vi "Cleanup.vi"(8 "error in (no error)":errorcluster, 11 "OBS in":refnum<class "OBS.lvclass">) -> (0 "error out":errorcluster)   [LabVIEW 2020, in "obs-websocket.lvlib" / "OBS.lvclass"]
uses:
  OBS.lvclass
  Command.ctl
  OBS.lvclass/OBS.ctl
  lv-promises/Promises/Promise/Promise.lvclass
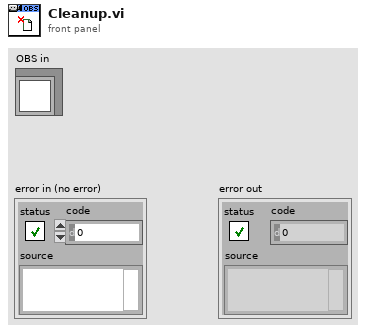
[diagram p1: front panel]
types:
  T1 = typedef "obs-websocket.lvlib/OBS.lvclass/Command.ctl" = enum16{"Open", "Close", "Stop"}
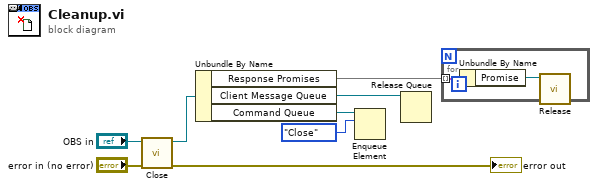
[diagram p0: block diagram]
diagram:
  n1 = call "Close.vi"("error in (no error)"="error in (no error)", "OBS in"="OBS in") -> ("error out"=→"error out":errorcluster, "OBS out"=w6:refnum<class "OBS.lvclass">)  [unwired: 8 in]
  n2 = Unbundle By Name(w6) -> ("Response Promises"=w1:map{string, refnum<class "Promise.lvclass">}, "Client Message Queue"=w5:refnum<queue>, "Command Queue"=w3:refnum<queue>)
  n3 = Enqueue Element(queue=w3, element=Command."Close") -> ()  [unwired: 2 in, 3 out]
  n4 = Release Queue(queue=w5) -> ()  [unwired: 2 in, 3 out]
  n5 = for {
    tunnel: w1 -> [w10] mode=indexing
    n6 = Unbundle By Name(w10) -> ("Promise"=w9:refnum<class "Promise.lvclass">)
    n7 = call "Release.vi"("Promise in"=w9) -> ()  [unwired: 11 in]
  }
